vi "Set Page Attribute.vi"(8 "error in (no error)":errorcluster, 10 "Pag Attribute":T1, 11 "QTab Class in":refnum<class "QTab Class.lvclass">) -> (0 "error out":errorcluster, 3 "QTab Class out":refnum<class "QTab Class.lvclass">)   [LabVIEW 2020, in "QTab.lvlib" / "QTab Class.lvclass"]
uses:
  QTab Class.lvclass
  Pag Attribute.ctl
  Command.ctl
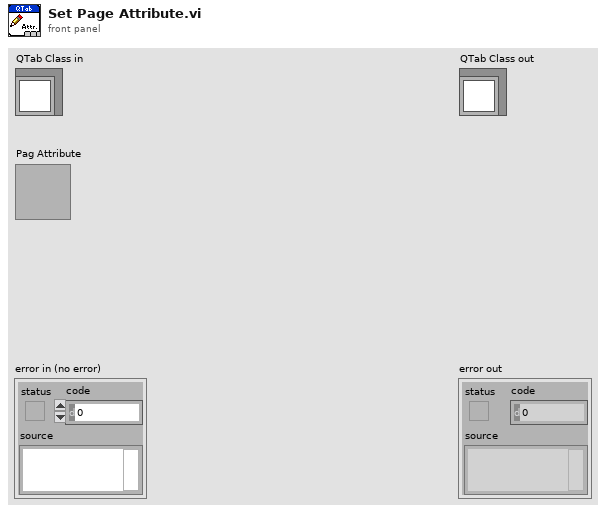
[diagram p1: front panel]
types:
  T1 = typedef "QTab.lvlib/QTab Class.lvclass/Pag Attribute.ctl" = cluster{"VI Refnum":refnum<vi>, "Page Name":string, "Closeable":bool, "Draggable":bool, "Pop-Out":bool}
  T2 = typedef "QTab.lvlib/QTab Class.lvclass/Command.ctl" = enum16{"Startup", "Add Page", "Close All Page", "Set Page Attribute", "Pop-out", "Merage", "Insert", "Stop"}
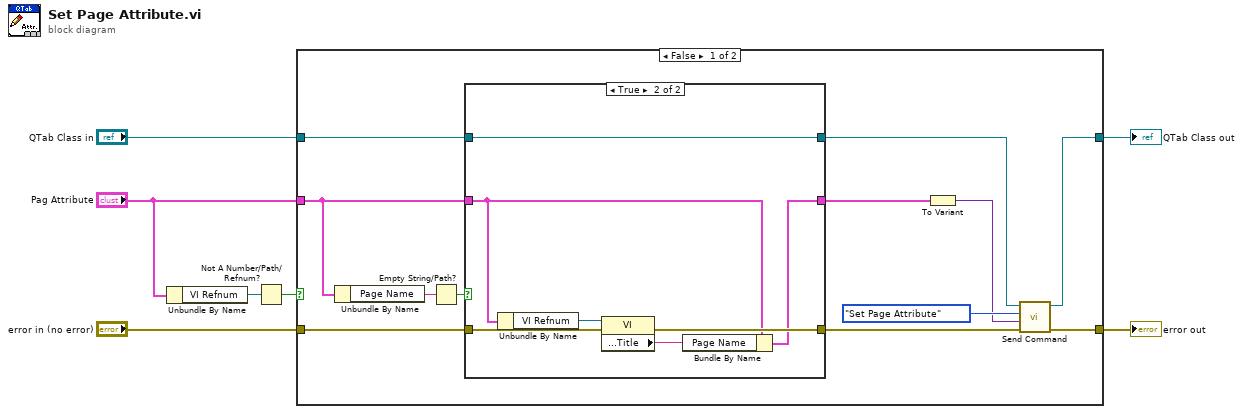
[diagram p0: block diagram]
diagram:
  n1 = Unbundle By Name("Pag Attribute") -> ("VI Refnum"=w6:refnum<vi>)
  n2 = Not A Number/Path/Refnum?(number/path/refnum=w6) -> (NaN/Path/Refnum?=w7:bool)
  n3 = case shown="False" w7 {
    tunnel: "error in (no error)" -> [w15 w30]
    tunnel: "QTab Class in" -> [w13 w31]
    tunnel: [w19 w31] -> w1
    tunnel: [w18 w30] -> w2
    tunnel: "Pag Attribute" -> [w10 _]
    frame False {
      n4 = Unbundle By Name(w10) -> ("Page Name"=w9:string)
      n5 = Empty String/Path?(string/path=w9) -> (empty?=w14:bool)
      n6 = case shown="True" w14 {
        tunnel: w15 -> [w21 w28]
        tunnel: w13 -> [w22 w29]
        tunnel: [w22 w29] -> w12
        tunnel: [w21 w27] -> w11
        tunnel: w10 -> [w20 w25]
        tunnel: [w20 w23] -> w8
        frame False {
        }
        frame True {
          n7 = Unbundle By Name(w25) -> ("VI Refnum"=w26:refnum<vi>)
          n8 = property class="VI"(reference=w26, error in=w28) -> (error out=w27:errorcluster, "Front Panel.Title"=w24:string)  [unwired: 1 out]
          n9 = Bundle By Name(cluster=w25, "Page Name"=w24) -> (w23:T1)
        }
      }
      n10 = To Variant(anything=w8) -> (Variant=w16:variant)
      n11 = call "Send Command.vi"("error in (no error)"=w11, "Data"=w16, "Command"=Command."Set Page Attribute", "QTab Class in"=w12) -> ("error out"=w18:errorcluster, "QTab Class out"=w19:refnum<class "QTab Class.lvclass">)  [unwired: 6 in]
    }
    frame True {
    }
  }
  "error out" <- w2
  "QTab Class out" <- w1
